vi "LJM logger read register list config.vi"(3 "Default Register List":string[](array[string])=["DAC0", "DAC1", "AIN_ALL_RESOLUTION_INDEX", "AIN_ALL_RANGE", "AIN0_NEGATIVE_CH", "AIN0_EF_INDEX", "AIN0_EF_CONFIG_A", "DIO4_EF_INDEX", "DIO4_EF_CONFIG_A", "DIO4_EF_ENABLE"], 4 "filename":string="expconfig.cfg", 5 "Working Directory":path) -> (0 "error out":errorcluster, 1 "Good Program Config":bool, 2 "Register List":string[](array[string]))   [LabVIEW 2026]
uses:
  <vilib>/Utility/config.llb/Read Key (String).vi
  <vilib>/Utility/config.llb/NI_LVConfig.lvlib
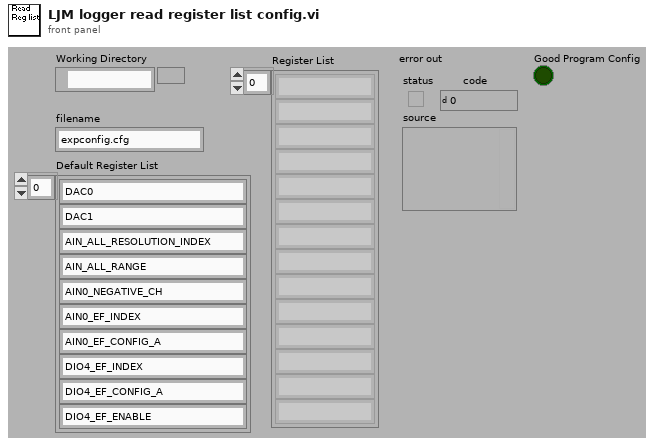
[diagram p1: front panel]
types:
  T1 = typedef "NI_LVConfig.lvlib/Config Data RefNum.ctl" = refnum<k1>
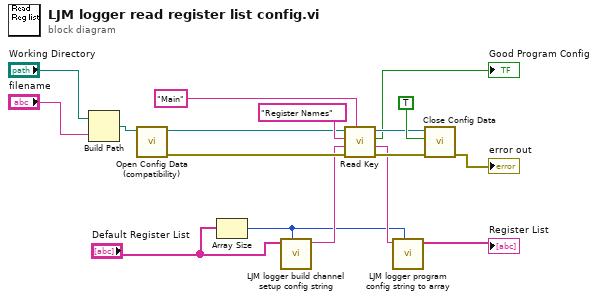
[diagram p0: block diagram]
diagram:
  n1 = Build Path(base path="Working Directory", name or relative path="filename") -> (appended path=w16:path)
  n2 = call <vilib>:"Open Config Data (compatibility).vi"("configuration file path"=w16) -> ("error out"=w10:errorcluster, "refnum"=w11:T1)  [unwired: 8 in, 1 out]
  n3 = Array Size(array="Default Register List") -> (size(s)=w2:i32)
  n4 = call "LJM logger build channel setup config string.vi"("Max Num Elements"=w2, "String list 1"="Default Register List") -> ("String 1 formatted"=w5:string)  [unwired: 6 in, 3 out]
  n5 = call-poly <vilib>:"Read Key.vi"("section"="Main", "error in (no error)"=w10, "default value"=w5, "key"="Register Names", "refnum"=w11) -> ("error out"=w7:errorcluster, "value"=w4:string, "found?"=→"Good Program Config":bool, "refnum out"=w8:T1)  [unwired: 3 in]
  n6 = call "LJM logger program config string to array.vi"("Max Num Elements"=w2, "String Config String In"=w4) -> ("String Config Array Out"=→"Register List":string[])  [unwired: 6 in, 3 out]
  n7 = call <vilib>:"Close Config Data.vi"("error in (no error)"=w7, "write file if changed (T)"=TRUE ("write configuration file? (F)"), "refnum"=w8) -> ("error out"=→"error out":errorcluster)  [unwired: 7 in, 1 out]
